vi "Update Motor State Value.vi"(8 "error in (no error)":errorcluster, 9 "state mode":T1 items=["undefined", "angle", "velocity"], 10 "value":dbl, 11 "motorcommunication in":refnum<class "NI_Robotics_Motor Communication Val.lvclass">) -> (0 "error out":errorcluster, 1 "failed?":bool, 3 "motor communication out":refnum<class "NI_Robotics_Motor Communication Val.lvclass">)   [LabVIEW 2017, in "NI_Robotics_Motor Communication Val.lvclass"]
uses:
  <vilib>/robotics/Actuation/Motor Communication Val/NI_Robotics_Motor Communication Val.lvclass
  <vilib>/robotics/Actuation/Motor Communication/Motor State Mode.ctl
  <vilib>/robotics/Actuation/Motor Communication Val/NI_Robotics_Motor Communication Val.lvclass/NI_Robotics_Motor Communication Val.ctl
  <vilib>/robotics/Actuation/Motor Communication/NI_Robotics_Motor Communication.lvclass
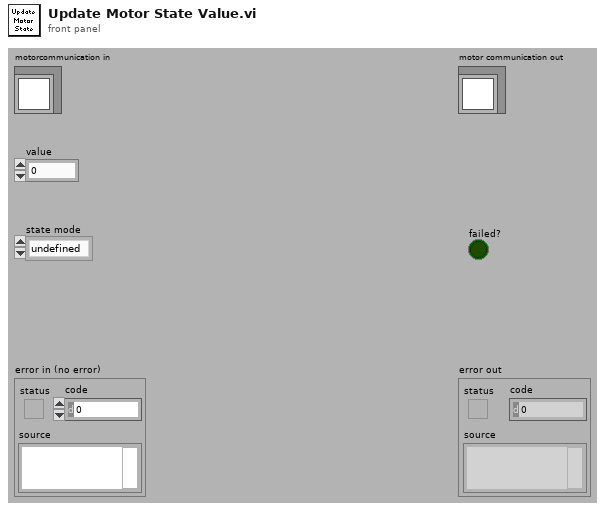
[diagram p1: front panel]
types:
  T1 = typedef "NI_Robotics_Motor Communication.lvclass/Motor State Mode.ctl" = u16
  T2 = typedef "NI_Robotics_Motor Communication.lvclass/Motor State Value.ctl" = cluster{"angle":dbl, "velocity":dbl, "state mode":T1}
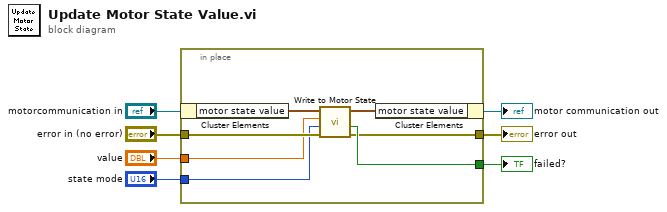
[diagram p0: block diagram]
diagram:
  n1 = in-place {
    in-place-border: [w13] -> w6
    in-place-border: "error in (no error)" -> [w12]
    in-place-border: "value" -> [w11]
    in-place-border: "state mode" -> [w10]
    in-place-border: [w9] -> w7
    n2 = in-place-cluster #1("motorcommunication in") -> ("motor state value"=w8:T2)
    n3 = call <vilib>:"Write to Motor State.vi"("error in (no error)"=w12, "state mode"=w10, "value"=w11, "motor state in"=w8) -> ("error out"=w9:errorcluster, "failed?"=w13:bool, "motor state out"=w14:T2)  [unwired: 5 in]
    n4 = in-place-cluster #1("motor state value"=w14) -> (→"motor communication out":refnum<class "NI_Robotics_Motor Communication Val.lvclass">)
  }
  "error out" <- w7
  "failed?" <- w6
